vi "Initialize.vi"(7 "Serial Configuration":T1={"Baud Rate"=9600, "Flow Control"=0, "Parity"=0, "Data Bits"=8} {"Flow Control" items=["NONE", "SOFTWARE"]; "Data Bits" items=["7"=7, "8"=8]; "Parity" items=["NONE", "ODD", "EVEN"]; "Baud Rate" items=["300"=300, "600"=600, "1200"=1200, "2400"=2400, "4800"=4800, "9600"=9600, "19200"=19200]}, 8 "error in (no error)":errorcluster, 9 "Reset (True)":bool=TRUE, 10 "ID Query (True)":bool=TRUE, 11 "VISA resource name":refnum<visa-resource-name>) -> (0 "error out":errorcluster, 3 "VISA resource name out":refnum<visa-resource-name>)   [LabVIEW 2025]
doc: "This VI passes the addressing information in the instrument decriptor to the Instr Open VI and returns the instrument ID. You can optionally reset the instrument by setting the front panel reset control. You must run this VI before using any of the instrument driver VIs for this instrument."
uses:
  <vilib>/ErrorRing/Error Ring.xnode
panel:
  # "true\n\nfalse"
  # "true\n\nfalse"
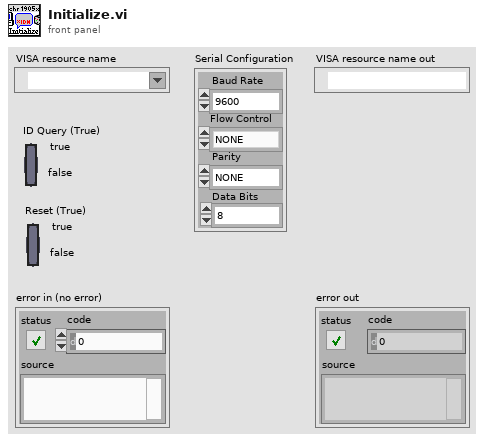
[diagram p1: front panel]
types:
  T1 = cluster{"Baud Rate":u32, "Flow Control":u16, "Parity":u16, "Data Bits":u16}
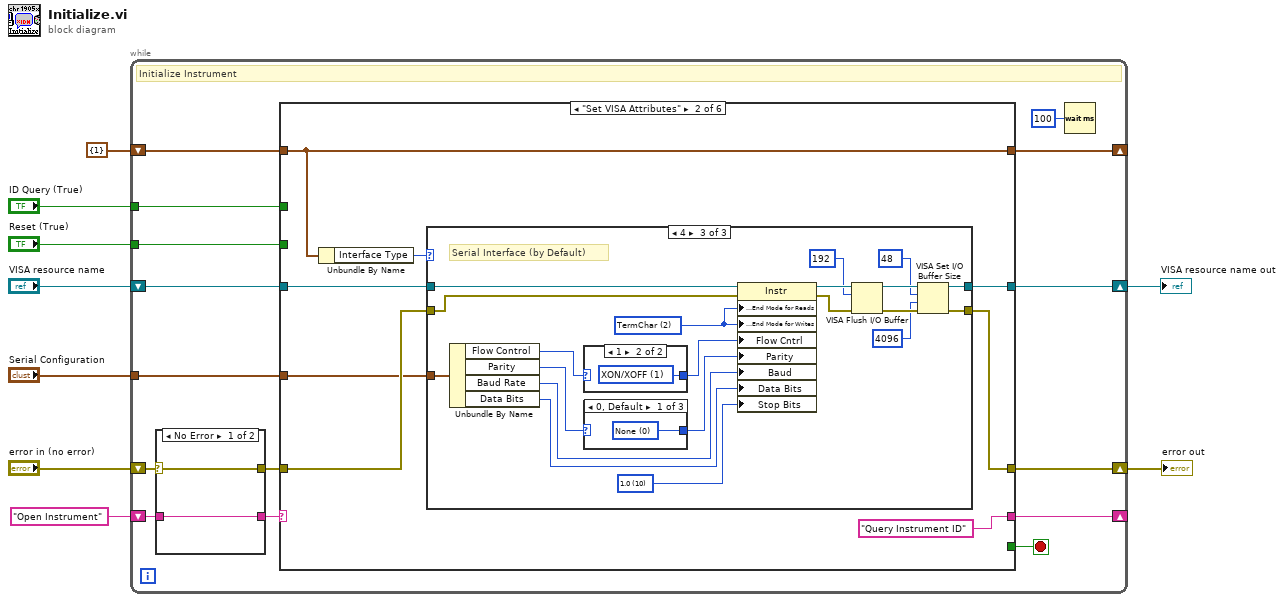
[diagram p0: block diagram]
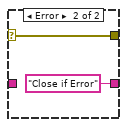
[diagram p2: hidden frame]
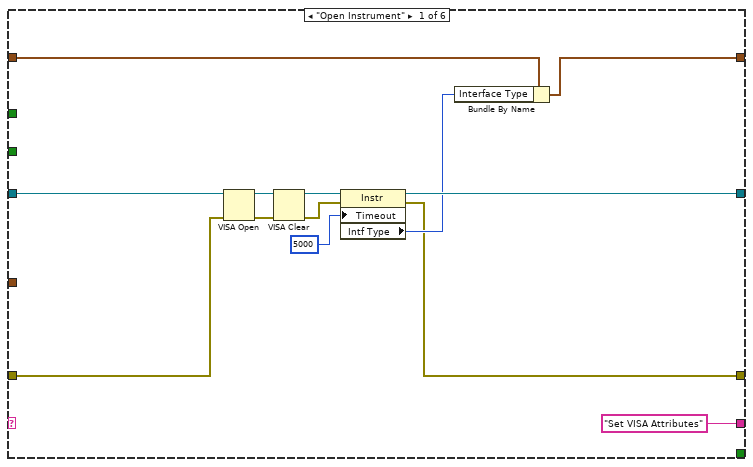
[diagram p3: hidden frame]
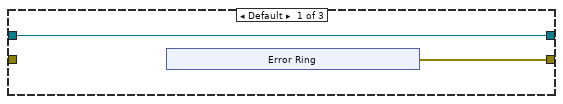
[diagram p4: hidden frame]
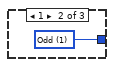
[diagram p6: hidden frame]
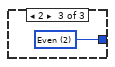
[diagram p7: hidden frame]
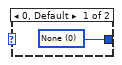
[diagram p8: hidden frame]
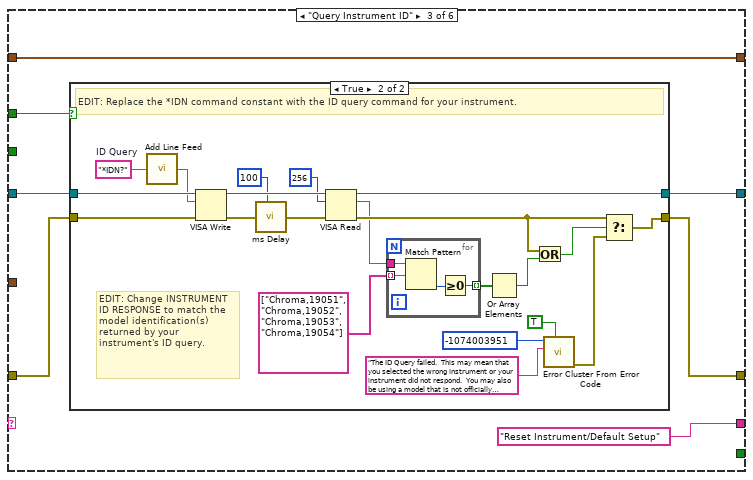
[diagram p9: hidden frame]
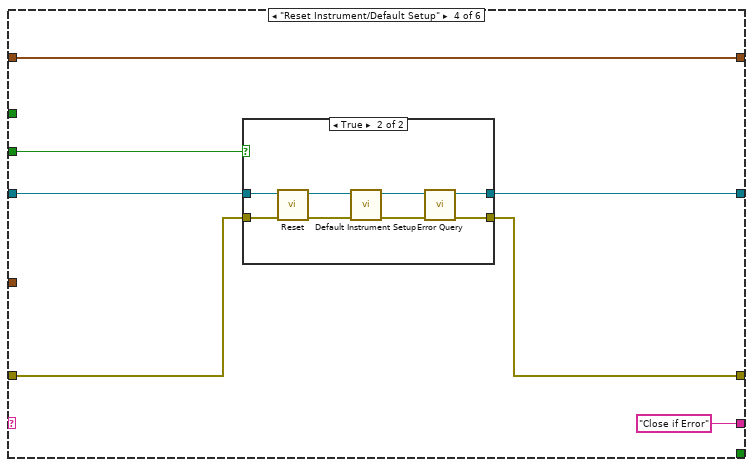
[diagram p11: hidden frame]
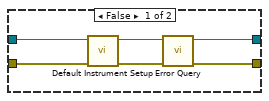
[diagram p12: hidden frame]
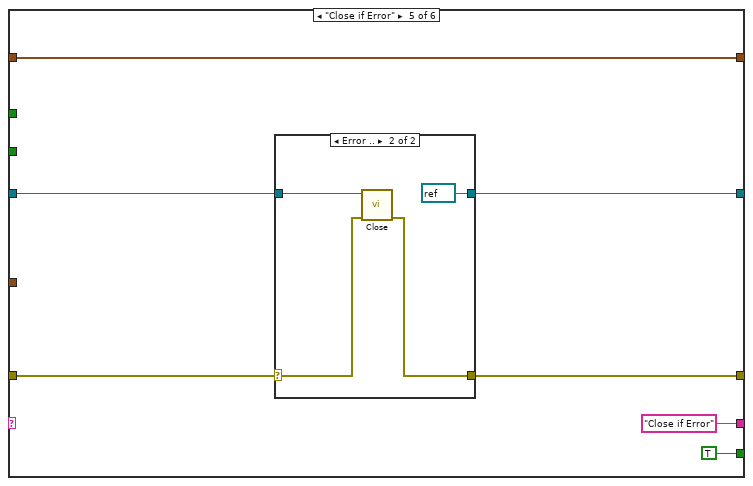
[diagram p13: hidden frame]
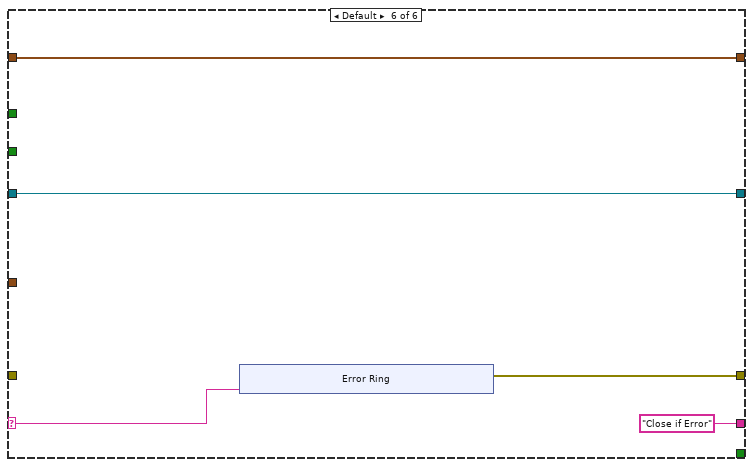
[diagram p15: hidden frame]
diagram:
  n1 = while {
    shift-right: [w23] -> _
    shift-left: cluster{"Interface Type":u16} {"Interface Type"=1} -> [w24]
    shift-right: [w22] -> _
    shift-left: "Open Instrument" -> [w15]
    shift-right: [w21] -> w1
    shift-left: "error in (no error)" -> [w17]
    tunnel: "Reset (True)" -> [w13]
    tunnel: "ID Query (True)" -> [w12]
    tunnel: "Serial Configuration" -> [w11]
    shift-right: [w20] -> w7
    shift-left: "VISA resource name" -> [w19]
    stop <- w18 stop-if-true
    # "Initialize Instrument"
    n2 = case shown="No Error" w17 {
      selector: w17 -> [w26 w28]
      tunnel: [w26 w28] -> w16
      tunnel: w15 -> [w25 _]
      tunnel: [w25 "Close if Error"] -> w14
      frame No Error {
      }
      frame Error {
      }
    }
    n3 = case shown="\"Set VISA Attributes\"" w14 {
      selector: w14 -> [_ _ _ _ _ w154]
      tunnel: w24 -> [w38 w49 w90 w124 w145 w156]
      tunnel: [w37 w49 w90 w124 w145 w156] -> w23
      tunnel: ["Set VISA Attributes" "Query Instrument ID" "Reset Instrument/Default Setup" "Close if Error" "Close if Error" "Close if Error"] -> w22
      tunnel: [w29 w42 w84 w118 w139 w153] -> w21
      tunnel: w16 -> [w39 w48 w88 w123 w142 _]
      tunnel: [w41 w47 w87 w121 w140 w155] -> w20
      tunnel: w19 -> [w34 w45 w89 w122 w141 w155]
      tunnel: [_ _ _ _ TRUE _] -> w18
      tunnel: w13 -> [_ _ _ w119 _ _]
      tunnel: w12 -> [_ _ w85 _ _ _]
      tunnel: w11 -> [_ w44 _ _ _ _]
      frame "Open Instrument" {
        n4 = VISA Open(error in (no error)=w39, VISA resource name=w34) -> (VISA resource name=w40:refnum<visa-resource-name>, error out=w35:errorcluster)  [unwired: 3 in]
        n5 = VISA Clear(VISA resource name=w40, error in (no error)=w35) -> (VISA resource name out=w33:refnum<visa-resource-name>, error out=w32:errorcluster)
        n6 = property class="Instr"(reference=w33, error in=w32, "Timeout"=u32 5000 ("Tmo Value")) -> (reference out=w41:refnum<visa-resource-name>, error out=w29:errorcluster, "Intf Type"=w30:u16)
        n7 = Bundle By Name(cluster=w38, "Interface Type"=w30) -> (w37:cluster{"Interface Type":u16})
      }
      frame "Set VISA Attributes" {
        n8 = Unbundle By Name(w49) -> ("Interface Type"=w43:u16)
        n9 = case shown="4" w43 {
          tunnel: [w51 w57 w62] -> w47
          tunnel: [w50 w58 w64] -> w42
          tunnel: w48 -> [_ w58 w77]
          tunnel: w45 -> [w51 w57 w78]
          tunnel: w44 -> [_ _ w67]
          frame Default {
            n10 = xnode "Error Ring"() -> ("error out"=w50:errorcluster)
          }
          frame 1 {
            # "GPIB when interface is intalled"
          }
          frame 4 {
            w59 = u16 10 items=["1.0"=10, "1.5"=15, "2.0"=20] ("Serial Settings:Stop Bits")
            w75 = u16 2 items=["None", "LastBit", "TermChar"] ("Serial Settings:Serial End Mode for Reads")
            # "Serial Interface (by Default)"
            n11 = Unbundle By Name(w67) -> ("Flow Control"=w74:u16, "Parity"=w73:u16, "Baud Rate"=w71:u32, "Data Bits"=w70:u16)
            n12 = case shown="1" w74 {
              tunnel: [w82 w83] -> w69
              frame 0, Default {
                w82 = u16 0 items=["None", "XON/XOFF", "RTS/CTS", "XON/XOFF & RTS/CTS", "DTR/DSR", "XON/XOFF & DTR/DSR"] ("Serial Settings:Flow Control")
              }
              frame 1 {
                w83 = u16 1 items=["None", "XON/XOFF", "RTS/CTS", "XON/XOFF & RTS/CTS", "DTR/DSR", "XON/XOFF & DTR/DSR"] ("Serial Settings:Flow Control")
              }
            }
            n13 = case shown="0, Default" w73 {
              tunnel: [w79 w80 w81] -> w72
              frame 0, Default {
                w79 = u16 0 items=["None", "Odd", "Even", "Mark", "Space"] ("Serial Settings:Parity")
              }
              frame 1 {
                w80 = u16 1 items=["None", "Odd", "Even", "Mark", "Space"] ("Serial Settings:Parity")
              }
              frame 2 {
                w81 = u16 2 items=["None", "Odd", "Even", "Mark", "Space"] ("Serial Settings:Parity")
              }
            }
            n14 = property class="Instr"(reference=w78, error in=w77, "Serial Settings:End Mode for Reads"=w75, "Serial Settings:End Mode for Writes"=w75, "Flow Cntrl"=w69, "Parity"=w72, "Baud"=w71, "Data Bits"=w70, "Stop Bits"=w59) -> (reference out=w76:refnum<visa-resource-name>, error out=w68:errorcluster)
            n15 = VISA Flush I/O Buffer(VISA resource name=w76, mask (16)=u16 192, error in (no error)=w68) -> (VISA resource name out=w63:refnum<visa-resource-name>, error out=w65:errorcluster)
            n16 = VISA Set I/O Buffer Size(VISA resource name=w63, mask (16)=u16 48, size (4096)=u32 4096, error in (no error)=w65) -> (VISA resource name out=w62:refnum<visa-resource-name>, error out=w64:errorcluster)
          }
        }
      }
      frame "Query Instrument ID" {
        n17 = case shown="True" w85 {
          tunnel: [w91 w112] -> w84
          tunnel: [w92 w109] -> w87
          tunnel: w89 -> [w92 w110]
          tunnel: w88 -> [w91 w111]
          frame False {
          }
          frame True {
            w94 = "*IDN?"  # ID Query
            # "EDIT: Change INSTRUMENT ID RESPONSE to match the model identification(s) returned by your instrument's ID query."
            # "EDIT: Replace the *IDN command constant with the ID query command for your instrument."
            n18 = call "Add Line Feed.vi"("Command string"=w94) -> ("Concatenated string"=w93:string)  [unwired: 4 in]
            n19 = VISA Write(VISA resource name=w110, write buffer=w93, error in (no error)=w111) -> (VISA resource name out=w113:refnum<visa-resource-name>, error out=w97:errorcluster)  [unwired: 1 out]
            n20 = call "ms Delay.vi"("miliseconds to wait"=u32 100 ("Time Delay [ms]"), "error in (no error)"=w97) -> ("error out"=w96:errorcluster)  [unwired: 6 in, 1 out]
            n21 = VISA Read(VISA resource name=w113, byte count=u32 256, error in (no error)=w96) -> (VISA resource name out=w109:refnum<visa-resource-name>, read buffer=w98:string, error out=w102:errorcluster)  [unwired: 1 out]
            n22 = for {
              tunnel: string[] ["Chroma,19051", "Chroma,19052", "Chroma,19053", "Chroma,19054"] -> [w114] mode=indexing
              tunnel: w98 -> [w116]
              tunnel: [w115] -> w101 mode=indexing
              n23 = Match Pattern(string=w116, regular expression=w114) -> (offset past match=w117:i32)  [unwired: 1 in, 3 out]
              n24 = Greater Or Equal To 0?(x=w117) -> (x >= 0?=w115:bool)
            }
            n25 = Or Array Elements(Boolean array=w101) -> (logical OR=w100:bool)
            n26 = Or(x=w102, y=w100) -> (x .or. y?=w99:bool)
            n27 = call <vilib>:"Error Cluster From Error Code.vi"("show call chain? (False)"=TRUE, "error message (\"\")"="The ID Query failed.  This may mean that you selected the wrong instrument or your instrument did not respond.  You may also be using a model that is not officially supported by this driver.  If you are sure that you have selected the correct instrument and it is responding, try disabling the ID Query." ("Source (VI Name)"), "error code (0)"=-1074003951 ("Code")) -> ("error out"=w108:errorcluster)  [unwired: 6 in]
            n28 = Select(t=w102, s=w99, f=w108) -> (s? t:f=w112:errorcluster)
          }
        }
      }
      frame "Reset Instrument/Default Setup" {
        n29 = case shown="True" w119 {
          tunnel: w123 -> [w130 w138]
          tunnel: [w128 w131] -> w118
          tunnel: w122 -> [w127 w137]
          tunnel: [w125 w132] -> w121
          frame False {
            n30 = call "Default Instrument Setup.vi"("error in (no error)"=w130, "VISA resource name"=w127) -> ("error out"=w129:errorcluster, "VISA resource name out"=w126:refnum<visa-resource-name>)  [unwired: 8 in]
            n31 = call "Error Query.vi"("error in (no error)"=w129, "VISA resource name"=w126) -> ("error out"=w128:errorcluster, "VISA resource name out"=w125:refnum<visa-resource-name>)  [unwired: 6 in, 2 out]
          }
          frame True {
            n32 = call "Reset.vi"("error in (no error)"=w138, "VISA resource name"=w137) -> ("error out"=w133:errorcluster, "VISA resource name out"=w134:refnum<visa-resource-name>)  [unwired: 8 in]
            n33 = call "Default Instrument Setup.vi"("error in (no error)"=w133, "VISA resource name"=w134) -> ("error out"=w136:errorcluster, "VISA resource name out"=w135:refnum<visa-resource-name>)  [unwired: 8 in]
            n34 = call "Error Query.vi"("error in (no error)"=w136, "VISA resource name"=w135) -> ("error out"=w131:errorcluster, "VISA resource name out"=w132:refnum<visa-resource-name>)  [unwired: 6 in, 2 out]
          }
        }
      }
      frame "Close if Error" {
        n35 = case shown="Error .." w142 {
          selector: w142 -> [w147 w149]
          tunnel: w141 -> [w146 w151]
          tunnel: [w146 refnum<visa-resource-name> refnum ("VISA resource name")] -> w140
          tunnel: [w147 w148] -> w139
          frame No Error {
          }
          frame Error {
            n36 = call "Close.vi"("error in (no error)"=w149, "VISA resource name"=w151) -> ("error out"=w148:errorcluster)  [unwired: 9 in]
          }
        }
      }
      frame Default {
        n37 = xnode "Error Ring"("parameter 0"=w154) -> ("error out"=w153:errorcluster)
      }
    }
    n38 = Wait (ms)(milliseconds to wait=u32 100) -> ()  [unwired: 1 out]
  }
  "VISA resource name out" <- w7
  "error out" <- w1
